vi "Write.vi"(8 "error in (no error)":errorcluster, 10 "Array":string[][](array[string]), 11 "CSV in":refnum<class "CSV.lvclass">) -> (0 "error out":errorcluster, 3 "CSV out":refnum<class "CSV.lvclass">)   [LabVIEW 2014, in "CSV.lvclass"]
uses:
  CSV.lvclass
  CSV.lvclass/CSV.ctl
  <vilib>/Utility/file.llb/Write To Spreadsheet File (string).vi
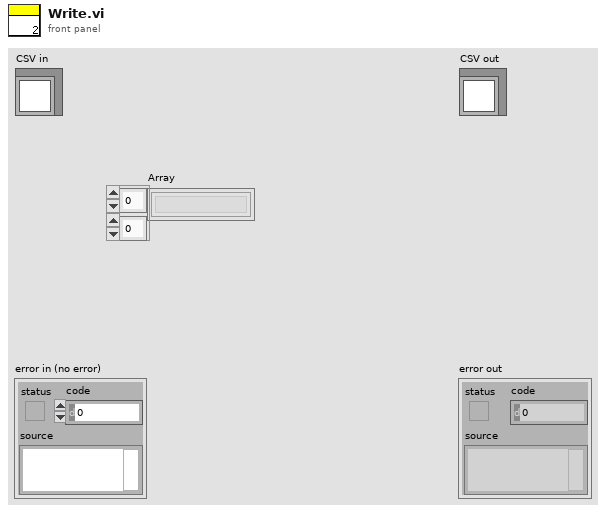
[diagram p1: front panel]
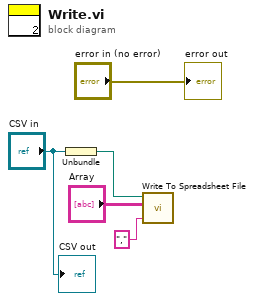
[diagram p0: block diagram]
diagram:
  n1 = Unbundle("CSV in") -> (w5:path)
  n2 = call-poly <vilib>:"Write To Spreadsheet File.vi"("delimiter (\\t)"=",", "2D data"="Array", "file path (dialog if empty)"=w5) -> ()  [unwired: 5 in, 1 out]
  "error out" <- "error in (no error)"
  "CSV out" <- "CSV in"
